vi "Init Graph.vi"(4 "Z Scale.Marker Values[]":cluster{"Numeric":dbl, "Numeric":u32}[](array[cluster]), 6 "X-Graph Ref":refnum<vi>, 7 "Y-Graph Ref":refnum<vi>, 8 "error in (no error)":errorcluster, 9 "Images Size":cluster{"Height":u32, "Width":u32}, 10 "IntGraph Ref":refnum<vi>, 11 "Intensity Graph in":refnum<class "TG Graph.lvclass">) -> (0 "error out":errorcluster, 3 "Intensity Graph out":refnum<class "TG Graph.lvclass">)   [LabVIEW 2023, in "TG Graph.lvclass"]
uses:
  TG Graph.lvclass
  TG Graph.lvclass/TG Graph.ctl
  TG Base Graph/TG Base Graph.lvclass
  D:/git/LabVIEW-Helpers/TG Graph Class/TG Base Graph/TG Base Graph.lvclass
  D:/git/LabVIEW-Helpers/TG Graph Class/TG Graph/TG Graph.lvclass
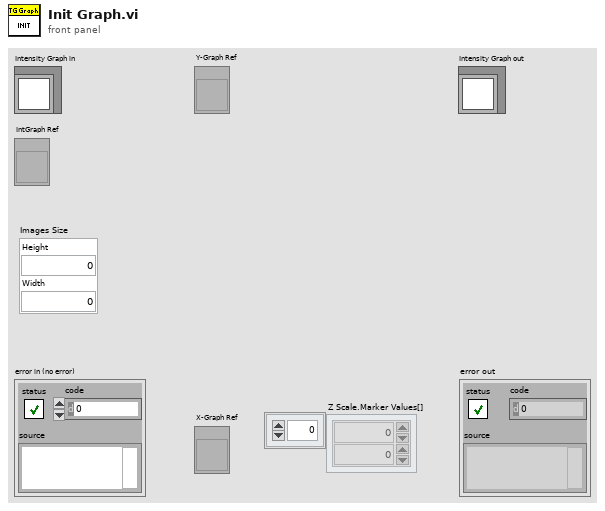
[diagram p1: front panel]
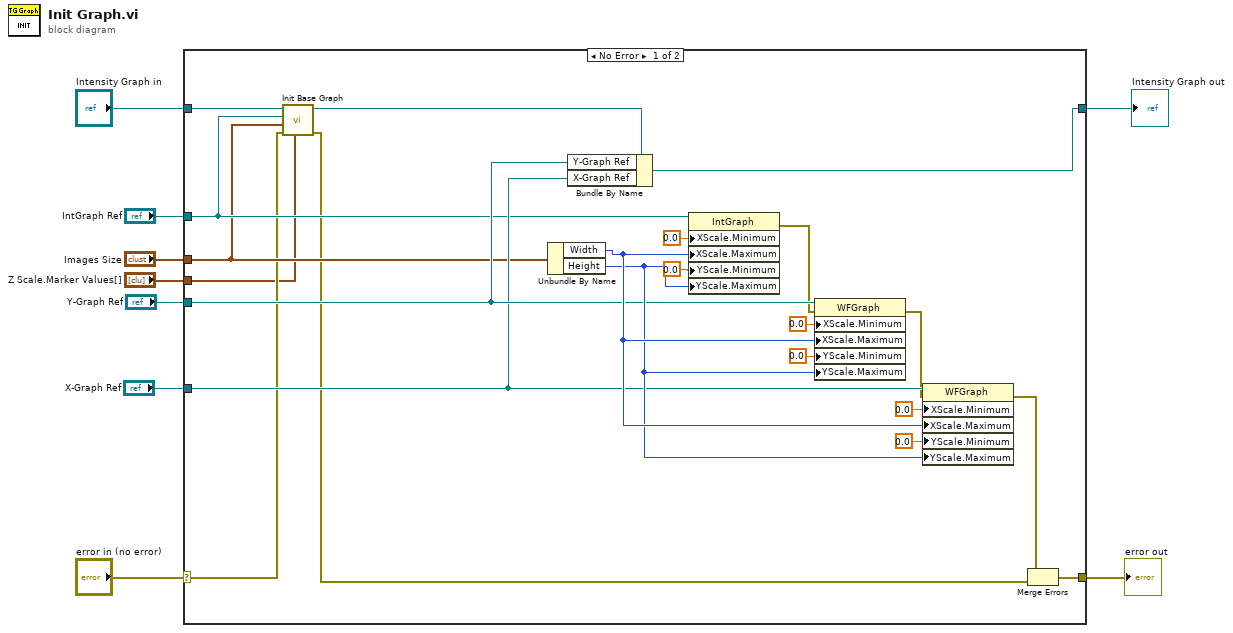
[diagram p0: block diagram]
diagram:
  n1 = case shown="No Error" "error in (no error)" {
    selector: "error in (no error)" -> [w12 w33]
    tunnel: [w21 w33] -> w8
    tunnel: [w20 w32] -> w6
    tunnel: "Intensity Graph in" -> [w16 w32]
    tunnel: "IntGraph Ref" -> [w14 _]
    tunnel: "Y-Graph Ref" -> [w23 _]
    tunnel: "X-Graph Ref" -> [w22 _]
    tunnel: "Images Size" -> [w13 _]
    tunnel: "Z Scale.Marker Values[]" -> [w11 _]
    frame No Error {
      n2 = call "Init Base Graph.vi"("Z Scale.Marker Values[]"=w11, "error in (no error)"=w12, "Sizes"=w13, "IntGraph Ref"=w14, "TG Base Graph in"=w16) -> ("error out"=w10:errorcluster, "TG Base Graph out"=w15:refnum<class "TG Graph.lvclass">)  [unwired: 5 in]
      n3 = Unbundle By Name(w13) -> ("Width"=w25:u32, "Height"=w24:u32)
      n4 = Bundle By Name(cluster=w15, "Y-Graph Ref"=w23, "X-Graph Ref"=w22) -> (w20:refnum<class "TG Graph.lvclass">)
      n5 = property class="IntGraph"(reference=w14, "XScale.Minimum"=0.0 ("X Scale.Range:Minimum"), "XScale.Maximum"=w25, "YScale.Minimum"=0.0 ("Y Scale.Range:Minimum"), "YScale.Maximum"=w24) -> (error out=w17:errorcluster)  [unwired: 1 in, 1 out]
      n6 = property class="WFGraph"(reference=w23, error in=w17, "XScale.Minimum"=0.0 ("X Scale.Range:Minimum"), "XScale.Maximum"=w25, "YScale.Minimum"=0.0 ("Y Scale.Range:Minimum"), "YScale.Maximum"=w24) -> (error out=w18:errorcluster)  [unwired: 1 out]
      n7 = property class="WFGraph"(reference=w22, error in=w18, "XScale.Minimum"=0.0 ("X Scale.Range:Minimum"), "XScale.Maximum"=w25, "YScale.Minimum"=0.0 ("Y Scale.Range:Minimum"), "YScale.Maximum"=w24) -> (error out=w19:errorcluster)  [unwired: 1 out]
      n8 = Merge Errors(w19, w10) -> (w21:errorcluster)
    }
    frame Error {
    }
  }
  "error out" <- w8
  "Intensity Graph out" <- w6
